vi "Unlock Report.vi"(2 "error in (no error)":errorcluster, 3 "Report Ref In":T1) -> (0 "error out":errorcluster, 1 "Report Ref Out":T1)   [LabVIEW 2013, in "XCel Report Engine.lvlib"]
doc: "Removes worksheet protection from all worksheets in the open Excel report.\n\nThis VI reverses the protection applied by Lock Report.vi and allows the workbook contents to be modified again. Calling it when the worksheets are already unprotected has no additional effect.\n\nThe password used by Lock Report.vi is not required to perform this operation."
uses:
  XCel Report Engine.lvlib
  C:/Users/m.santucci/Documents/ChatGPT/LV_REPORT_ENGINE/LV/DotNet/XCelReportEngine.dll
  LV/DotNet/XCelReportEngine.dll
  Controls/Report Ref.ctl
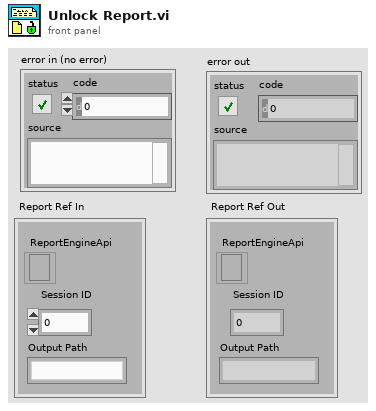
[diagram p1: front panel]
types:
  T1 = typedef "XCel Report Engine.lvlib/Report Ref.ctl" = cluster{"Session ID":i32, "Output Path":string, "ReportEngineApi":refnum<k24>}
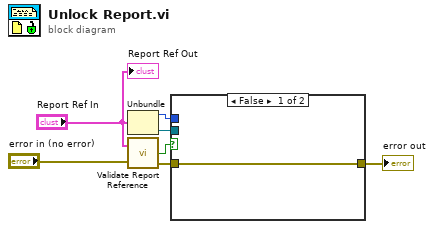
[diagram p0: block diagram]
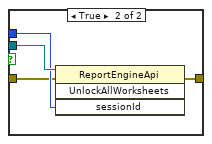
[diagram p2: hidden frame]
diagram:
  n1 = Unbundle("Report Ref In") -> ("Session ID"=w5:i32, "ReportEngineApi"=w7:refnum<k24>)  [unwired: 1 out]
  n2 = call "Validate Report Reference.vi"("Report Ref In"="Report Ref In", "error in (no error)"="error in (no error)") -> ("Valid"=w1:bool, "error out"=w2:errorcluster)  [unwired: 1 out]
  n3 = case shown="False" w1 {
    tunnel: w7 -> [_ w12]
    tunnel: [w8 w11] -> w6
    tunnel: w5 -> [_ w10]
    tunnel: w2 -> [w8 w9]
    frame False {
    }
    frame True {
      n4 = invoke class="ReportEngineApi" method="UnlockAllWorksheets"(reference=w12, error in=w9, "sessionId"=w10) -> (error out=w11:errorcluster)  [unwired: 1 in, 3 out]
    }
  }
  "error out" <- w6
  "Report Ref Out" <- "Report Ref In"
